vi "VI Revision Info.vi"(8 "error in (no error)":errorcluster, 11 "Path":path) -> (0 "error out":errorcluster, 3 "Latest Rev comment":string)   [LabVIEW 2018]
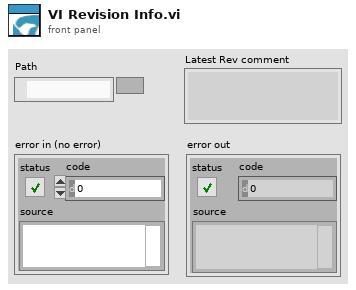
[diagram p1: front panel]
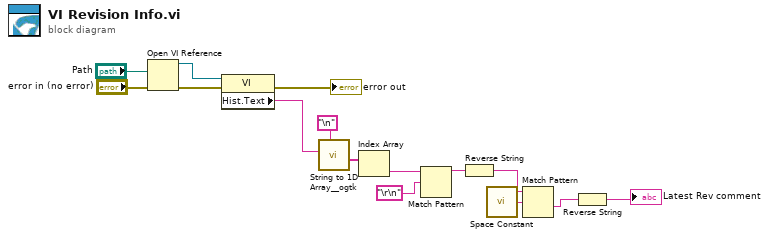
[diagram p0: block diagram]
diagram:
  n1 = Open VI Reference(vi path="Path", error in (no error)="error in (no error)") -> (vi reference=w12:refnum<vi>, error out=w13:errorcluster)  [unwired: 4 in]
  n2 = property class="VI"(reference=w12, error in=w13) -> (error out=→"error out":errorcluster, "Hist.Text"=w8:string)  [unwired: 1 out]
  n3 = call <userlib>:"String to 1D Array__ogtk.vi"("delimiter (Tab)"="\n", "string"=w8) -> ("Array of Strings"=w9:string[])  [unwired: 9 in]
  n4 = Index Array(array=w9) -> (element=w7:string)  [unwired: 1 in]
  n5 = Match Pattern(string=w7, regular expression="\r\n") -> (before substring=w5:string)  [unwired: 1 in, 3 out]
  n6 = Reverse String(1:w5) -> (0:w4:string)
  n7 = call <vilib>:"Space Constant.vi"() -> ("String"=w3:string)
  n8 = Match Pattern(string=w4, regular expression=w3) -> (after substring=w1:string)  [unwired: 1 in, 3 out]
  n9 = Reverse String(1:w1) -> (0:→"Latest Rev comment":string)
